vi "MB ICPCON Registers Manager Close.vi"(8 "error in":errorcluster, 11 "Data Reference":T1) -> (0 "error out":errorcluster)   [LabVIEW 2019, in "ICPCON Registers.lvlib"]
uses:
  ICPCON Registers.lvlib
  Ctl/ICPCON Data.ctl
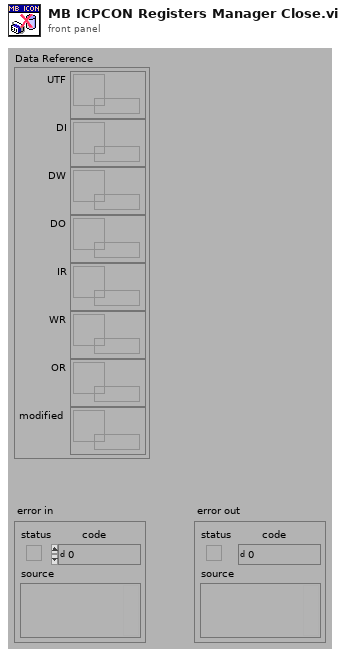
[diagram p1: front panel]
types:
  T1 = typedef "ICPCON Registers.lvlib/ICPCON Data.ctl" = cluster{"UTF":refnum<data-value>, "DI":refnum<data-value>, "DW":refnum<data-value>, "DO":refnum<data-value>, "IR":refnum<data-value>, "WR":refnum<data-value>, "OR":refnum<data-value>, "modified":refnum<data-value>}
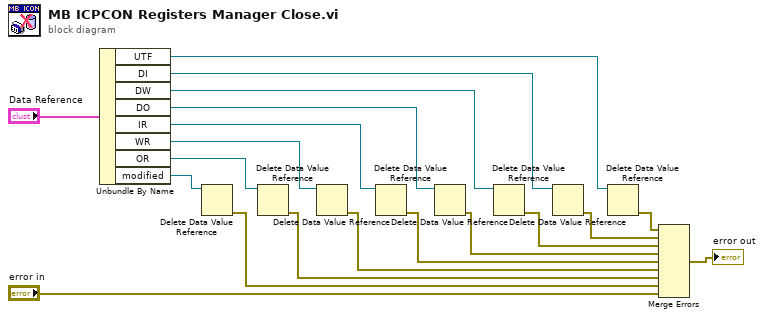
[diagram p0: block diagram]
diagram:
  n1 = Unbundle By Name("Data Reference") -> ("UTF"=w5:refnum<data-value>, "DI"=w19:refnum<data-value>, "DW"=w18:refnum<data-value>, "DO"=w17:refnum<data-value>, "IR"=w16:refnum<data-value>, "WR"=w9:refnum<data-value>, "OR"=w8:refnum<data-value>, "modified"=w2:refnum<data-value>)
  n2 = Delete Data Value Reference(data value reference=w2) -> (error out=w1:errorcluster)  [unwired: 1 in, 1 out]
  n3 = Delete Data Value Reference(data value reference=w8) -> (error out=w10:errorcluster)  [unwired: 1 in, 1 out]
  n4 = Delete Data Value Reference(data value reference=w9) -> (error out=w11:errorcluster)  [unwired: 1 in, 1 out]
  n5 = Delete Data Value Reference(data value reference=w16) -> (error out=w13:errorcluster)  [unwired: 1 in, 1 out]
  n6 = Delete Data Value Reference(data value reference=w17) -> (error out=w14:errorcluster)  [unwired: 1 in, 1 out]
  n7 = Delete Data Value Reference(data value reference=w18) -> (error out=w15:errorcluster)  [unwired: 1 in, 1 out]
  n8 = Delete Data Value Reference(data value reference=w19) -> (error out=w7:errorcluster)  [unwired: 1 in, 1 out]
  n9 = Delete Data Value Reference(data value reference=w5) -> (error out=w6:errorcluster)  [unwired: 1 in, 1 out]
  n10 = Merge Errors(w6, w7, w15, w14, w13, w11, w10, w1, "error in") -> (→"error out":errorcluster)
